vi "Remove names.vi"(10 "Array in":string[](array[string])) -> (2 "Array out":string[](array[string]))   [LabVIEW 2014]
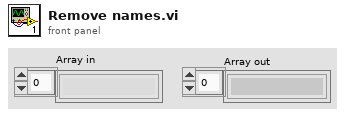
[diagram p1: front panel]
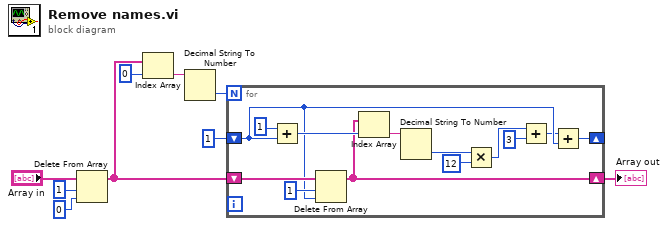
[diagram p0: block diagram]
diagram:
  n1 = Delete From Array(array="Array in", length=1, index=0) -> (array with subset deleted=w1:string[])  [unwired: 1 out]
  n2 = Index Array(array=w1, index=0) -> (element=w7:string)
  n3 = Decimal String To Number(string=w7) -> (number=w6:i32)  [unwired: 2 in, 1 out]
  n4 = for {
    N: w6 -> [_]
    shift-right: [w12] -> _
    shift-left: 1 ("index") -> [w13]
    shift-right: [w10] -> w3
    shift-left: w1 -> [w15]
    n5 = Add(x=1 ("index"), y=w13) -> (x+y=w16:i32)
    n6 = Delete From Array(array=w15, length=1, index=w13) -> (array with subset deleted=w10:string[])  [unwired: 1 out]
    n7 = Index Array(array=w10, index=w16) -> (element=w21:string)
    n8 = Decimal String To Number(string=w21) -> (number=w20:i32)  [unwired: 2 in, 1 out]
    n9 = Multiply(x=w20, y=12) -> (x*y=w18:i32)
    n10 = Add(x=w18, y=3) -> (x+y=w11:i32)
    n11 = Add(x=w11, y=w13) -> (x+y=w12:i32)
  }
  "Array out" <- w3
